vi "Data_aq.vi"() -> ()   [LabVIEW 2016]
doc: "Use this template to measure or generate signals using the DAQ Assistant Express VI and NI-DAQmx. Double click the DAQ Assistant Express VI to launch a configuration wizard which steps you through configuring a measurement or generation.\n\nNote: You must have an NI-DAQmx compatible device installed to use this Express VI. Refer to the DAQ Quick Start Guide for NI-DAQ 7.0 for a list of compatible devices."
uses:
  <vilib>/Platform/TimedLoop/XDataNode/timing_clust.ctl
  <vilib>/Platform/TimedLoop/XDataNode/nitl_modes.ctl
  <vilib>/Platform/TimedLoop/XDataNode/wakeup.ctl
  <vilib>/Platform/TimedLoop/XDataNode/loadnilvce.vi
  <vilib>/express/express shared/transition.llb/Dynamic To Waveform Array.vi
  <vilib>/express/express signal manip/GetorSetDDTAttributes/Set DDT Attributes/SetT0.vi
  <vilib>/express/express shared/transition.llb/Waveform Array To Dynamic.vi
  <vilib>/Utility/file.llb/Write Delimited Spreadsheet (string).vi
  <vilib>/Utility/file.llb/Write Delimited Spreadsheet (DBL).vi
  <vilib>/Platform/TimedLoop/XDataNode/XDataNode.xnode
  <vilib>/express/express signal manip/GetorSetDDTAttributes/Set DDT Attributes/Set DDT Properties.xnode
  <vilib>/Platform/TimedLoop/XDataNode/XDNodeRunTimeDep.lvlib
  <resource>/objmgr/ni.var.rc
panel:
  out "NH4 Probe":refnum<k21>="ni.var.io://localhost/Mod6/AI0"
  out "Na Probe":refnum<k21>="ni.var.io://localhost/Mod6/AI1"
  out "new file path (Not A Path if cancelled)":path
  in  "File Name:":string
  out "Saving?":bool
  out "Headers":string[](array[string])
  out "error out":errorcluster
  out "Na Live":dbl format="%#_4g"
  out "String 6":string="Na"
  in  "error in":errorcluster
  out "NH4 Live":dbl format="%#_4g"
  out "All data":dbl[][](array[numeric]) format="%#3.4f"
  out "current sample":dbl format="%#_3g"
  out "Time":string="K"
  out "Date":string="K"
  out "iter number":i32
  out "String 2":string="NH4"
  in  "stop":bool
  # "Live"
  # "Last 50"
  # "Last 100"
  # "All"
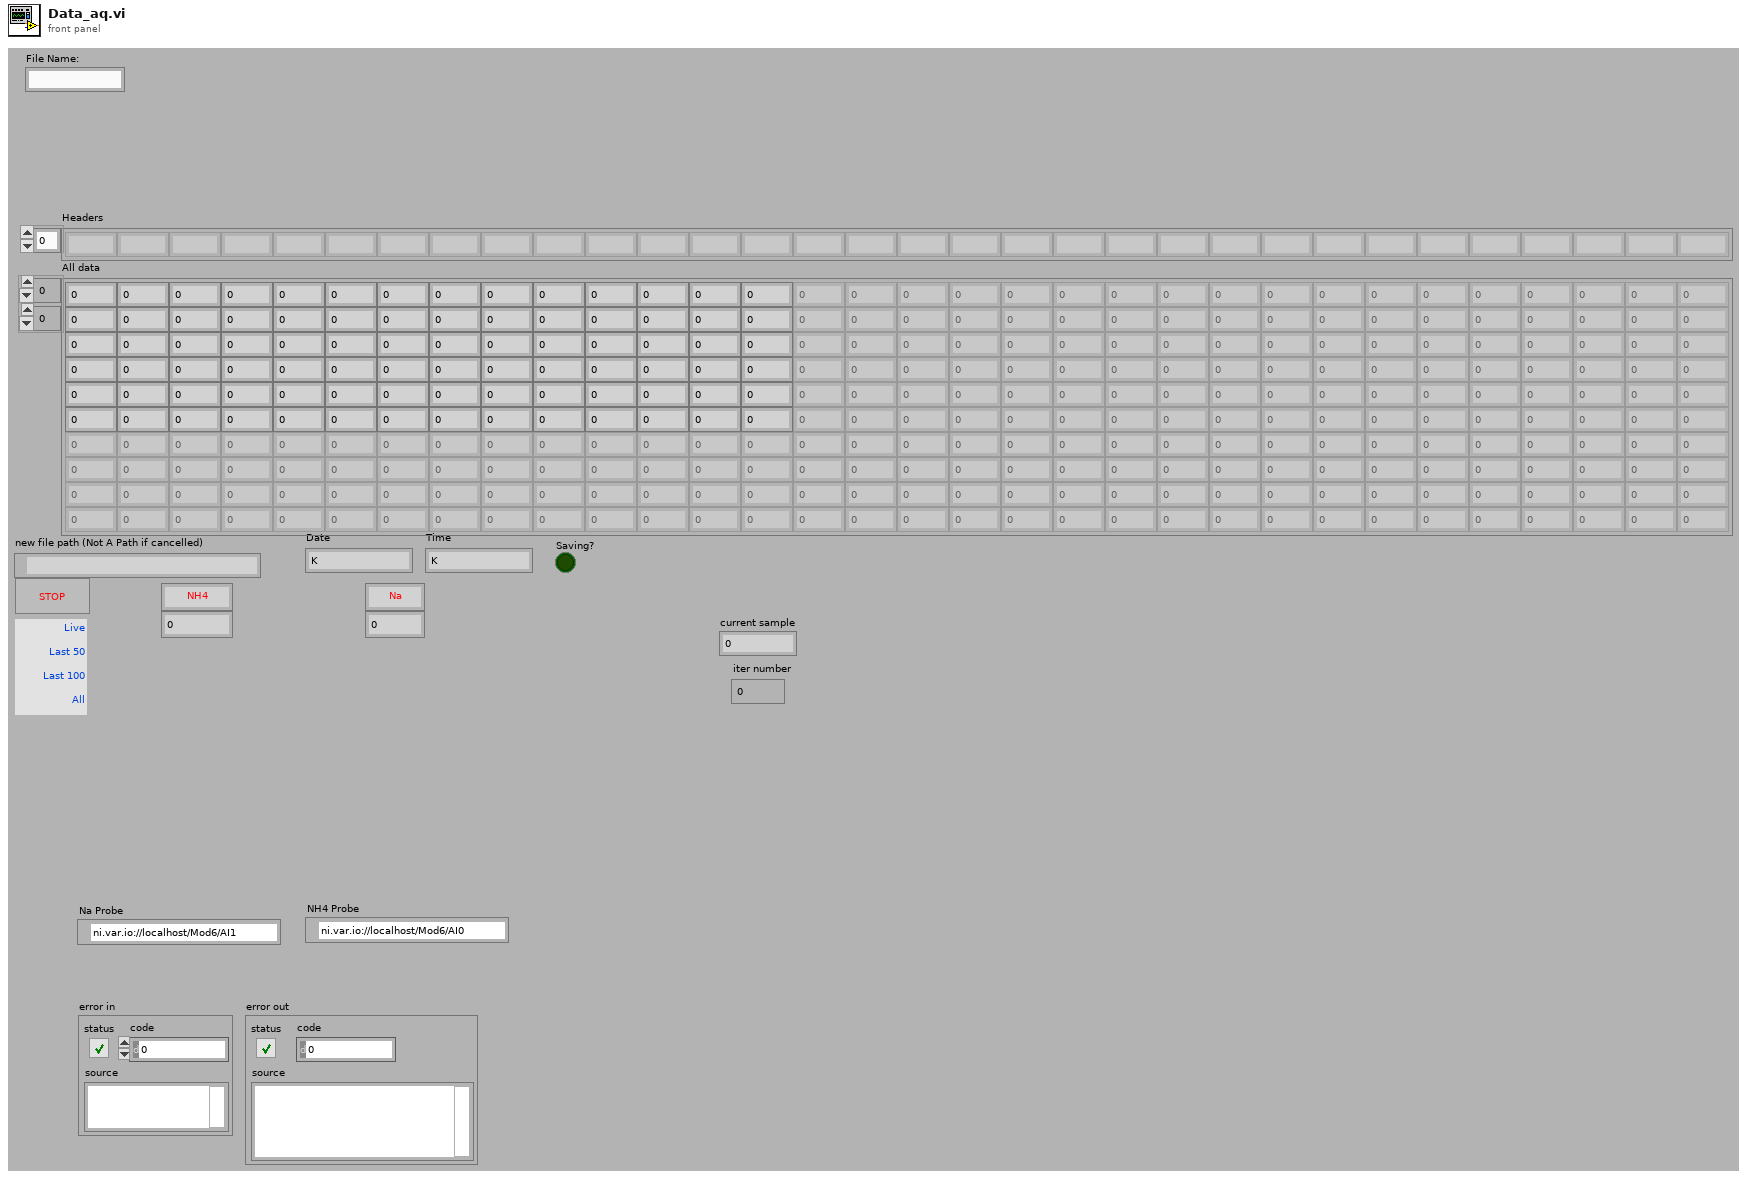
[diagram p1: front panel]
types:
  T1 = enum16{"open", "replace", "create", "open or create", "replace or create", "replace or create with confirmation"}
  T2 = typedef "XDNodeRunTimeDep.lvlib/timing_clust.ctl" = cluster{"Expected End [f-1]":u64, "Actual End [f-1]":u64, "Finished Late? [f-1]":bool, "Expected End [i-1]":u64, "Actual End [i-1]":u64, "Finished Late? [i-1]":bool, "Expected Start [i]":u64, "Actual Start [i]":u64, "Expected Start [f]":u64, "Actual Start [f]":u64, "Source Name":string, "Structure Name":string, "Period":i64, "Deadline":i64, "Offset":i64, "Start":i64, "Priority":i32, "Timeout":i32, "Mode":T3, "Wakeup Reason":T4, "Error":errorcluster, "Source Type":string, "Secondary Source Type":string, "Global End Time":u64, "Global Start Time":u64, "Frame Duration":u64, "Iteration Duration":u64, "Assigned CPU":i32, "I/O Scan Engine Mode":u32}
  T3 = typedef "XDNodeRunTimeDep.lvlib/nitl_modes.ctl" = enum32{"No Change", "Process missed periods, maintain original phase", "Discard missed periods, maintain original phase", "Process missed periods, ignore original phase", "Discard missed periods, ignore original phase"}
  T4 = typedef "XDNodeRunTimeDep.lvlib/wakeup.ctl" = enum32{"Normal", "Aborted", "Asynchronous wakeup", "Timing source error", "Timed loop error", "Timeout"}
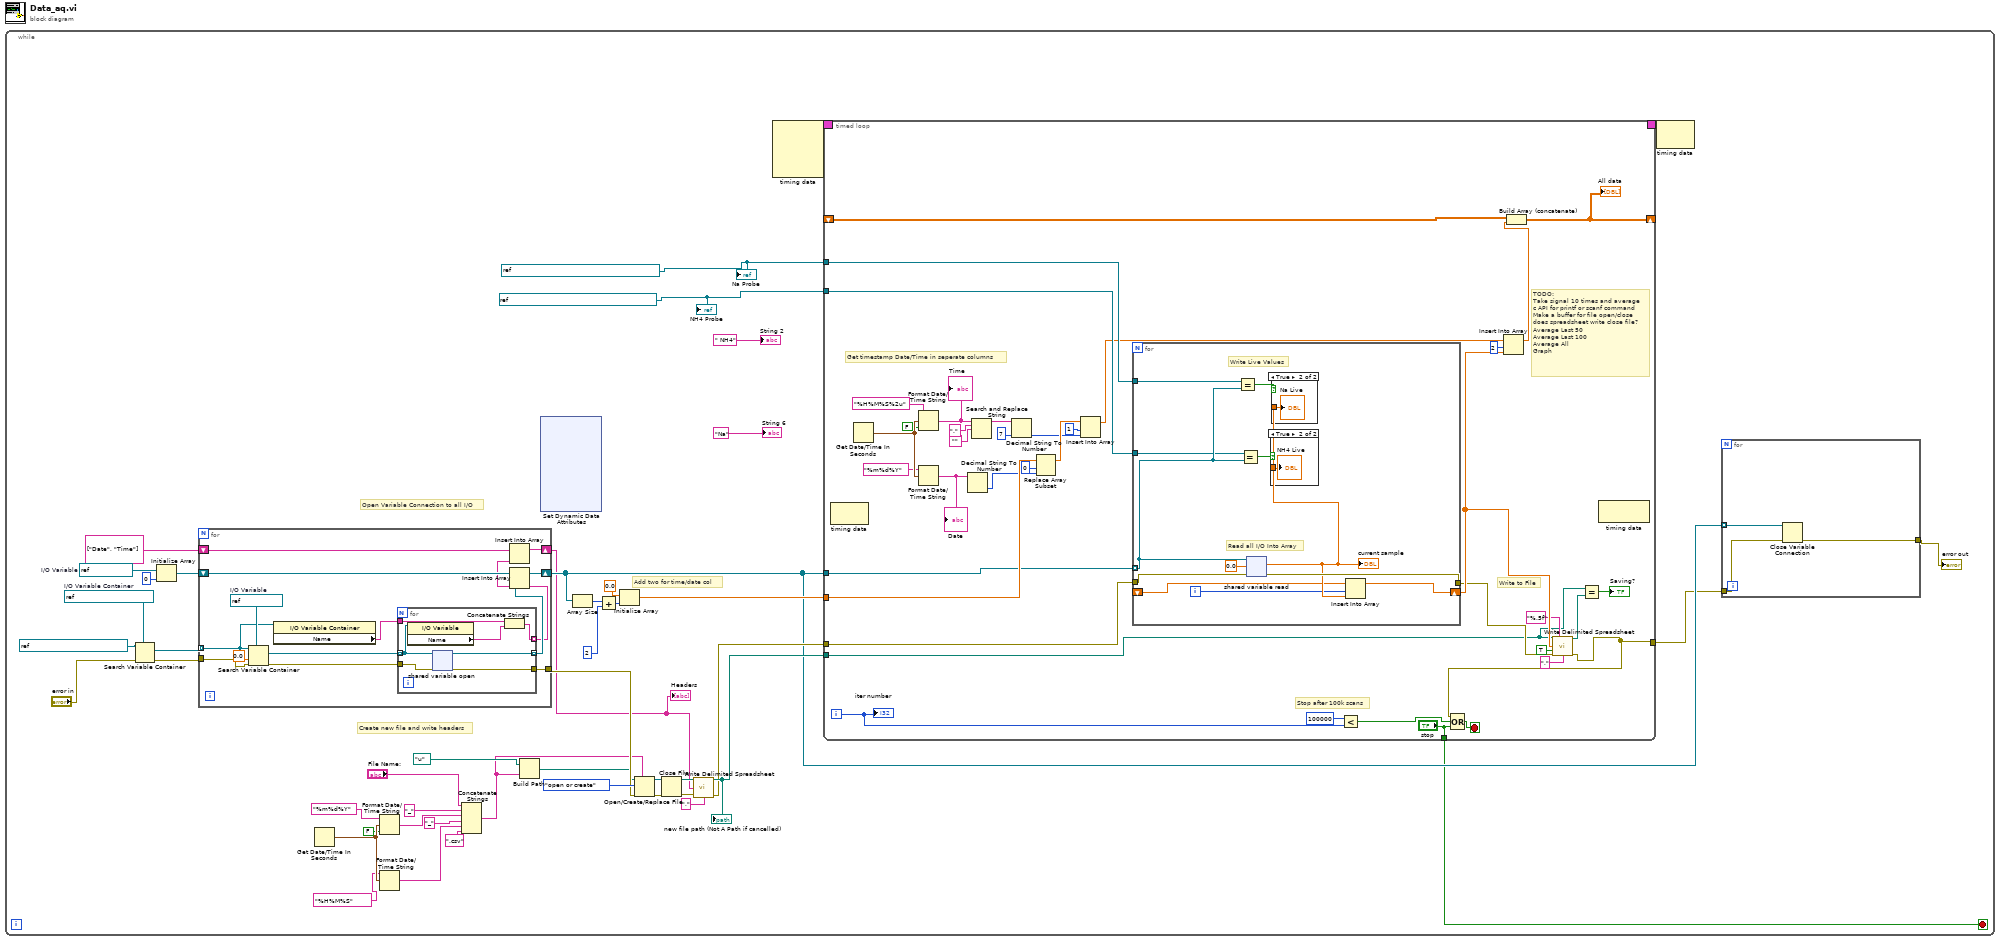
[diagram p0: block diagram]
diagram:
  n1 = while {
    stop <- w2 stop-if-true
    w15 = refnum<k21> "ni.var.io://localhost/Mod6/AI1" ("Variable Name Control/Indicator")
    w14 = refnum<k21> "ni.var.io://localhost/Mod6/AI0" ("Variable Name Control/Indicator")
    w40 = refnum<k21> refnum  # I/O Variable
    w43 = refnum<k21> refnum  # I/O Variable Container
    # "Create new file and write headers"
    # "Add two for time/date col"
    # "Open Variable Connection to all I/O"
    n2 = Search Variable Container(7:w43, 8:"error in", 11:refnum<k21> "ni.var.io://crio1-winklerlab" ("Variable Name Control/Indicator")) -> (0:w42:errorcluster, 2:w44:refnum<k21>[])  [unwired: 3 in, 1 out]
    n3 = Initialize Array(w40, 0 ("dimension size")) -> (w41:refnum<k21>[])
    n4 = for {
      tunnel: w44 -> [w123] mode=indexing
      tunnel: w42 -> [w132]
      shift-right: [w128] -> w22
      shift-left: w41 -> [w129]
      tunnel: [w127] -> w24
      shift-right: [w125] -> w18
      shift-left: string[] ["Date", "Time"] -> [w126]
      w135 = refnum<k21> refnum  # I/O Variable
      n5 = Search Variable Container(7:w135, 8:w132, 9:0.0, 11:w123) -> (0:w131:errorcluster, 2:w134:refnum<k21>[])  [unwired: 2 in, 1 out]
      n6 = property class="I/O Variable Container"(reference=w123) -> ("Name"=w122:string)  [unwired: 1 in, 2 out]
      n7 = for {
        tunnel: w134 -> [w139] mode=indexing
        tunnel: w131 -> [w142]
        tunnel: [w141] -> w130 mode=indexing
        tunnel: [w140] -> w127
        tunnel: [w136] -> w124 mode=indexing
        tunnel: w122 -> [w137]
        n8 = property class="I/O Variable"(reference=w139) -> ("Name"=w138:string)  [unwired: 1 in, 2 out]
        n9 = shared-variable-open(w139, w142) -> (w141:refnum<k21>, w140:errorcluster)  [unwired: 1 in]
        n10 = Concatenate Strings(w137, w138) -> (w136:string)
      }
      n11 = Insert Into Array(array=w126, new element=w124) -> (w125:string[])  [unwired: 1 in]
      n12 = Insert Into Array(array=w129, new element=w130) -> (w128:refnum<k21>[])  [unwired: 1 in]
    }
    "Headers" <- w18
    n13 = Get Date/Time In Seconds() -> (seconds since 1Jan1904=w12:timestamp)
    n14 = Format Date/Time String(time format string (%c)="%m%d%Y", seconds (now)=w12, UTC format=FALSE) -> (date/time string=w9:string)
    n15 = Format Date/Time String(time format string (%c)="%H%M%S", seconds (now)=w12) -> (date/time string=w5:string)  [unwired: 1 in]
    n16 = Concatenate Strings("File Name:", "_" ("string"), w9, "_" ("string"), w5, ".csv" ("string")) -> (w4:string)
    n17 = Build Path(base path=path "u:/" ("Save to:"), name or relative path=w4) -> (appended path=w16:path)
    n18 = xnode "Set Dynamic Data Attributes"() -> ()  [unwired: 4 in, 2 out]
    n19 = Array Size(array=w22) -> (size(s)=w36:i32)
    n20 = Add(x=w36, y=2) -> (x+y=w34:i32)
    n21 = Initialize Array(0.0, w34) -> (w37:dbl[])
    n22 = Open/Create/Replace File(file path (use dialog)=w16, error in=w24, prompt=w4, operation (0:open)=T1."open or create") -> (refnum out=w29:refnum<file>, error out=w30:errorcluster)  [unwired: 2 in, 1 out]
    n23 = Close File(refnum=w29, error in=w30) -> (path=w28:path, error out=w25:errorcluster)
    n24 = call-poly <vilib>:"Write Delimited Spreadsheet.vi"("file path (dialog if empty)"=w28, "1D data"=w18, "error in (no error)"=w25, "delimiter (\\t)"="," ("delimiter (\\t)")) -> ("new file path (Not A Path if cancelled)"=w27:path, "error out"=w23:errorcluster)  [unwired: 10 in]
    "new file path (Not A Path if cancelled)" <- w27
    n25 = node-c288() -> (w47:T2)  [unwired: 4 in]
    n26 = timed-loop {
      timing: w47 -> [_]
      timing-out: [_] -> w46
      tunnel: w22 -> [w86]
      tunnel: w37 -> [w93]
      tunnel: w23 -> [w103]
      tunnel: w27 -> [w70]
      tunnel: w15 -> [w87]
      tunnel: w14 -> [w88]
      shift-right: [w83] -> _
      shift-left: _ -> [w84]
      tunnel: [w68] -> w21
      tunnel: ["stop"] -> w2
      i -> [w85]
      stop <- w90 stop-if-true
      # "TODO: \nTake signal 10 times and average\nc API for printf or scanf command\nMake a buffer for file open/close \ndoes spreadsheet write close file?\nAverage Last 50\nAverage Last 100\nAverage All\nGraph"
      # "Stop after 100k scans"
      # "Write to File"
      # "Get timestamp Date/Time in seperate columns"
      n27 = node-c288() -> ()  [unwired: 1 in, 1 out]
      n28 = Get Date/Time In Seconds() -> (seconds since 1Jan1904=w101:timestamp)
      n29 = Format Date/Time String(time format string (%c)="%H%M%S%2u", seconds (now)=w101, UTC format=FALSE) -> (date/time string=w97:string)
      "Time" <- w97
      n30 = Format Date/Time String(time format string (%c)="%m%d%Y", seconds (now)=w101) -> (date/time string=w81:string)  [unwired: 1 in]
      "Date" <- w81
      n31 = Decimal String To Number(string=w81) -> (number=w80:i32)  [unwired: 2 in, 1 out]
      n32 = Search and Replace String(input string=w97, search string=".", replace string="") -> (result string=w96:string)  [unwired: 5 in, 3 out]
      n33 = Decimal String To Number(string=w96, default (0L)=7) -> (number=w79:i32)  [unwired: 1 in, 1 out]
      n34 = Replace Array Subset(array=w93, new element=w80, index=0) -> (w92:dbl[])
      n35 = Insert Into Array(array=w92, index=1, new element=w79) -> (w78:dbl[])
      n36 = for {
        tunnel: w86 -> [w113] mode=indexing
        tunnel: w103 -> [w115]
        shift-right: [w106] -> w75
        shift-left: _ -> [w107]
        tunnel: [w114] -> w73
        tunnel: w88 -> [w112]
        tunnel: w87 -> [w110]
        i -> [w104]
        # "Read all I/O Into Array"
        # "Write Live Values"
        n37 = Equal?(x=w110, y=w113) -> (x = y?=w108:bool)
        n38 = Equal?(x=w112, y=w113) -> (x = y?=w109:bool)
        n39 = shared-variable-read(w113, w115, 0.0) -> (w114:errorcluster, w111:dbl)  [unwired: 2 out]
        "current sample" <- w111
        n40 = case shown="True" w109 {
          tunnel: w111 -> [_ w117]
          frame False {
          }
          frame True {
            "NH4 Live" <- w117
          }
        }
        n41 = case shown="True" w108 {
          tunnel: w111 -> [_ w116]
          frame False {
          }
          frame True {
            "Na Live" <- w116
          }
        }
        n42 = Insert Into Array(array=w107, index=w104, new element=w111) -> (w106:dbl[])
      }
      n43 = Less?(x=100000, y=w85) -> (x < y?=w89:bool)
      n44 = Insert Into Array(array=w78, index=2, new element=w75) -> (w76:dbl[])
      n45 = Build Array (concatenate)(w84, w76) -> (w83:dbl[][])
      "All data" <- w83
      n46 = call-poly <vilib>:"Write Delimited Spreadsheet.vi"("file path (dialog if empty)"=w70, "format (%.3f)"="%.5f", "1D data"=w75, "append to file? (new file:F)"=TRUE, "error in (no error)"=w73, "delimiter (\\t)"="," ("delimiter (\\t)")) -> ("new file path (Not A Path if cancelled)"=w71:path, "error out"=w68:errorcluster)  [unwired: 8 in]
      n47 = Compound Arithmetic op=OR(w68, w89, "stop") -> (w90:bool)
      n48 = Equal?(x=w70, y=w71) -> (x = y?=→"Saving?":bool)
      n49 = node-c288() -> ()  [unwired: 1 in, 1 out]
      "iter number" <- w85
    }
    n50 = node-c288(w46) -> ()  [unwired: 1 out]
    n51 = for {
      tunnel: w22 -> [w50] mode=indexing
      tunnel: w21 -> [w49]
      tunnel: [w48] -> w20
      n52 = Close Variable Connection(8:w49, 11:w50) -> (0:w48:errorcluster)
    }
    "error out" <- w20
    "String 2" <- " NH4"
    "String 6" <- "Na"
    "Na Probe" <- w15
    "NH4 Probe" <- w14
  }
